vi "Get description.vi"(1 "Builder in":refnum<class "Builder.lvclass">) -> (3 "Applications":T1[](array[typedef]))   [LabVIEW 2025, in "App-Builder Library.lvlib" / "Builder.lvclass"]
uses:
  Builder.lvclass
  App descriptions.ctl
  Build Type.ctl
  Builder.lvclass/Builder.ctl
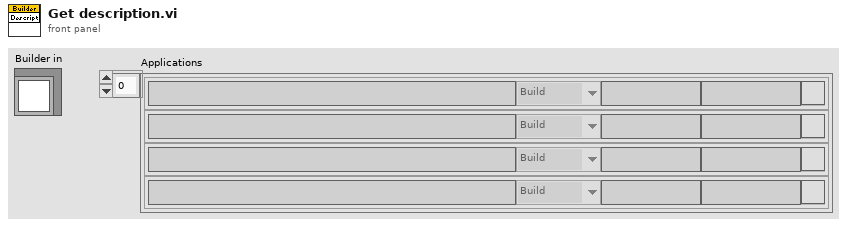
[diagram p1: front panel]
types:
  T1 = typedef "App-Builder Library.lvlib/Builder.lvclass/App descriptions.ctl" = cluster{"App Name":string, "Build Type":T2, "Current Version":string, "Next Version":string, "Check":bool}
  T2 = typedef "App-Builder Library.lvlib/Builder.lvclass/Build Type.ctl" = enum16{"Major", "Minor", "Fix", "Build"}
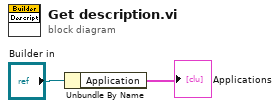
[diagram p0: block diagram]
diagram:
  n1 = Unbundle By Name("Builder in") -> ("Application"=→"Applications":T1[])
